vi "test Get Attached Channels.vi"(11 "Test Case In":refnum<class "Test PCANBasic.lvclass">) -> (0 "error out":errorcluster, 3 "Test Case Out":refnum<class "Test PCANBasic.lvclass">)   [LabVIEW 2020, in "Test PCANBasic.lvclass"]
uses:
  Test PCANBasic.lvclass
  C:/Program Files/National Instruments/LabVIEW 2026/vi.lib/Astemes/LUnit/Test Case.lvclass
  <vilib>/Astemes/LUnit/Test Case.lvclass/Test Case.ctl
  <vilib>/Astemes/LUnit/Test Case.lvclass
  source/PCANBasic.lvlib
  source/Get Attached Channels.vi
  source/PCAN Type.ctl
  source/TPCANHandle.ctl
  source/TPCANChannelInformation.ctl
panel:
  out "Channels":T1[](array[typedef]) {"PCAN Type" items=["Undefined"=0, "PCAN-ISA 82C200"=1, "PCAN-Dongle 82C200"=2, "PCAN-Dongle EPP82C200"=3, "PHYTEC ISA"=4, "PCAN-Dongle SJA1000"=5, "PCAN-Dongle EPP SJA 10000"=6, "PCAN-ISA SJA1000"=9]; "TPCANHandle" items=["PCAN_NONEBUS"=0, "PCAN_USBBUS1"=81, "PCAN_USBBUS2"=82, "PCAN_USBBUS3"=83, "PCAN_USBBUS4"=84, "PCAN_USBBUS5"=85, "PCAN_USBBUS6"=86, "PCAN_USBBUS7"=87, "PCAN_USBBUS8"=88, "PCAN_USBBUS9"=1289, "PCAN_USBBUS10"=1290, "PCAN_USBBUS11"=1291, "PCAN_USBBUS12"=1292, "PCAN_USBBUS13"=1293, "PCAN_USBBUS14"=1294, "PCAN_USBBUS15"=1295, "PCAN_USBBUS16"=1296]}
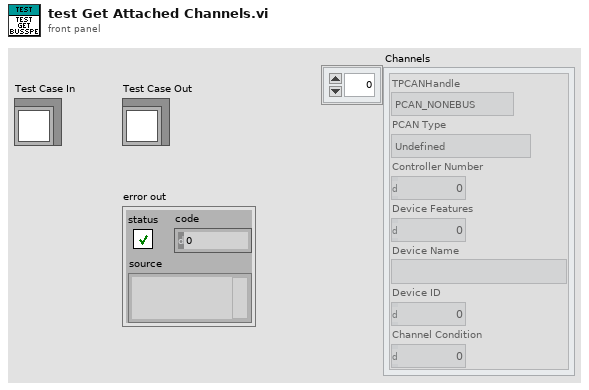
[diagram p1: front panel]
types:
  T1 = typedef "PCANBasic.lvlib/TPCANChannelInformation.ctl" = cluster{"TPCANHandle":T2, "PCAN Type":T3, "Controller Number":u8, "Device Features":u32, "Device Name":string, "Device ID":u32, "Channel Condition":u32}
  T2 = typedef "PCANBasic.lvlib/TPCANHandle.ctl" = u16
  T3 = typedef "PCANBasic.lvlib/PCAN Type.ctl" = u8
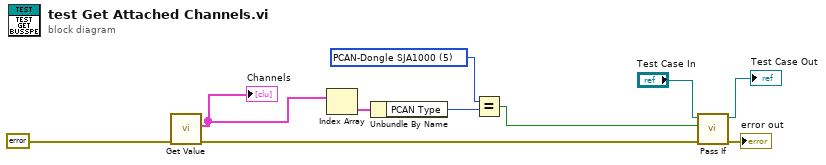
[diagram p0: block diagram]
diagram:
  w2 = T3 5 items=["Undefined"=0, "PCAN-ISA 82C200"=1, "PCAN-Dongle 82C200"=2, "PCAN-Dongle EPP82C200"=3, "PHYTEC ISA"=4, "PCAN-Dongle SJA1000"=5, "PCAN-Dongle EPP SJA 10000"=6, "PCAN-ISA SJA1000"=9] ("PCAN Type")
  n1 = call-poly "Get Value.vi"("error in"=errorcluster {"status"=FALSE, "code"=0, "source"=""}) -> ("error out"=w7:errorcluster, "Channels"=w5:T1[])  [unwired: 8 in, 1 out]
  "Channels" <- w5
  n2 = Index Array(array=w5) -> (element=w4:T1)  [unwired: 1 in]
  n3 = Unbundle By Name(w4) -> ("PCAN Type"=w3:T3)
  n4 = Equal?(x=w2, y=w3) -> (x = y?=w1:bool)
  n5 = call <vilib>:"Pass If.vi"("error in (no error)"=w7, "Pass?"=w1, "LUnit Test Case In"="Test Case In") -> ("error out"=→"error out":errorcluster, "LUnit Test Case Out"=→"Test Case Out":refnum<class "Test PCANBasic.lvclass">)  [unwired: 7 in]
